vi "Page - Bank.vi"(8 "error in (no error)":errorcluster, 11 "Node Ptr":T1 format="%.0x") -> (0 "error out":errorcluster)   [LabVIEW 2015, in "SLSC-12201 DIO System Explorer.lvlib"]
uses:
  SLSC-12201 DIO System Explorer.lvlib
  <vilib>/NI Veristand/Custom Device API/Custom Device Item Ref.ctl
  Shared/Constants.vi
  <vilib>/NI Veristand/Custom Device API/Get Item Property (Boolean).vi
  <vilib>/NI Veristand/Custom Device API/Custom Device API.lvlib
  Shared/SLSC-12201 DIO Shared.lvlib
panel:
  in  "*Enable Pull-up Resistors":bool
  in  "*33V Input Threshold":dbl caption="Input Threshold"
  in  "*5V Input Threshold":dbl caption="Input Threshold"
  in  "*Enable 5V Range":bool
  in  "*Select Vsup":u16(ring) caption="Voltage Supply Selector" items=["Off", "Vsup_0", "Vsup_1"]
  in  "SHDocVw.IWebBrowser2":refnum<k7>(container)
  in  "Header":cluster{"Section Name":string}={"Section Name"="Custom Device Item Settings"}
  in  "Description":string
  out "Name":string
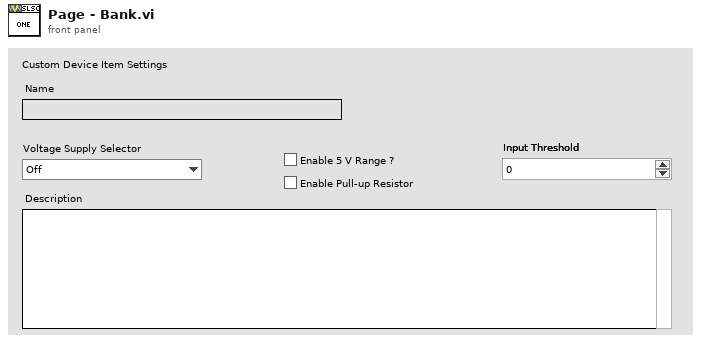
[diagram p1: front panel]
types:
  T1 = typedef "Custom Device API.lvlib/Custom Device Item Ref.ctl" = u64
  T2 = typedef "Custom Device API.lvlib/Custom Device Item Info.ctl" = cluster{"Name":string, "Is Channel":bool, "GUID":string, "Is Waveform":bool}
  T3 = typedef "Custom Device API.lvlib/Custom Device Channel.ctl" = cluster{"Type":T4, "Units":string, "Default Value":dbl, "Faultable":bool, "Scalable":bool}
  T4 = typedef "Custom Device API.lvlib/Custom Device Channel Type.ctl" = enum16{"Input", "Output"}
  T5 = cluster{"Channel Name":string, "SLSC Name":string, "Channel":T3}[]
  T6 = typedef "Custom Device API.lvlib/Custom Device Commands.ctl" = enum16{"Default", "Item renamed", "Shutdown", "Dynamic button pressed"}
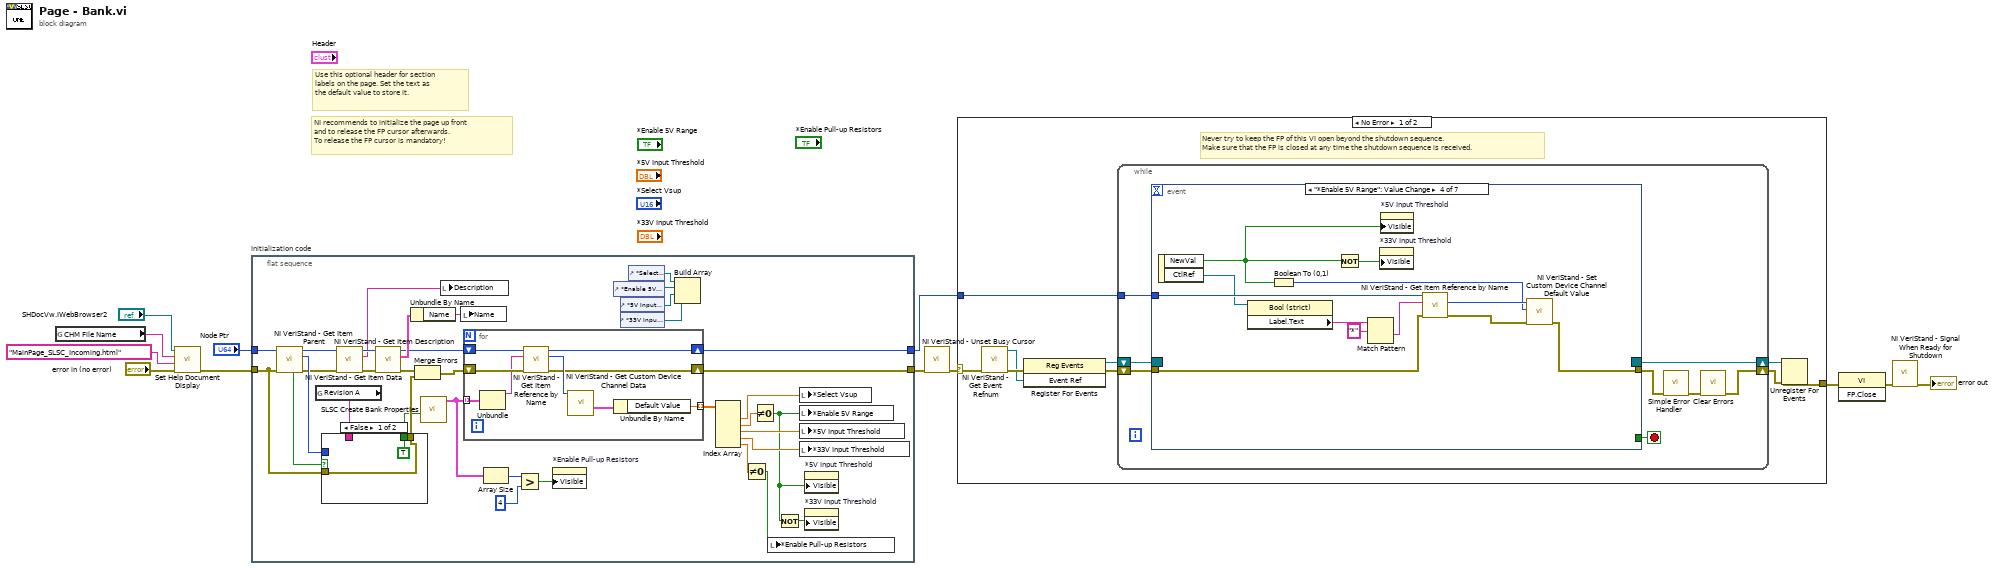
[diagram p0: block diagram]
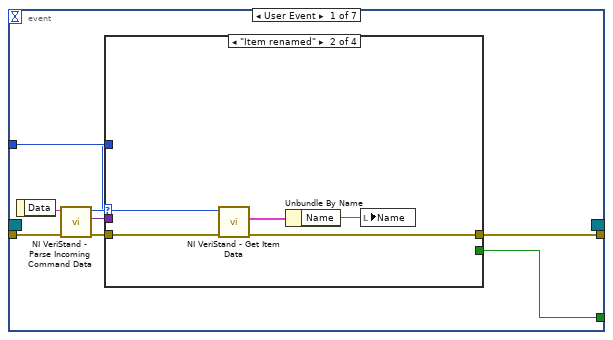
[diagram p2: hidden frame]
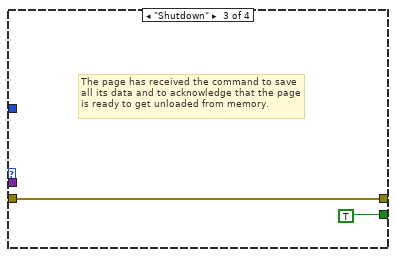
[diagram p4: hidden frame]
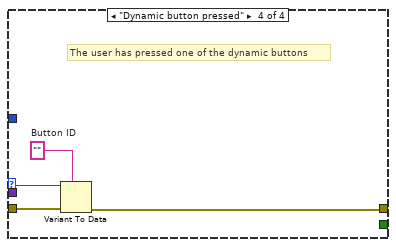
[diagram p5: hidden frame]
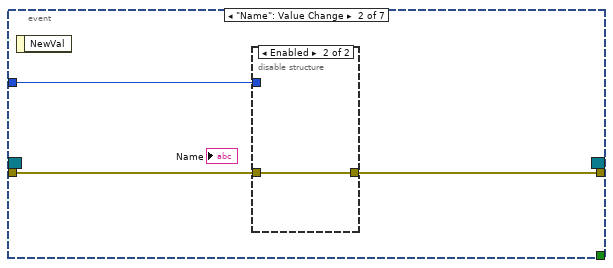
[diagram p6: hidden frame]
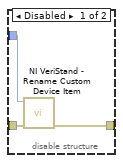
[diagram p7: hidden frame]
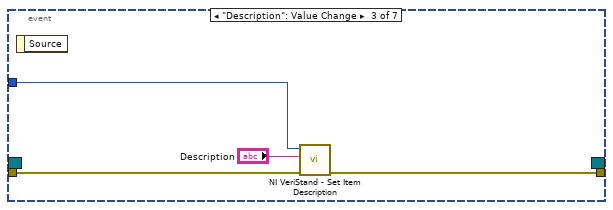
[diagram p8: hidden frame]
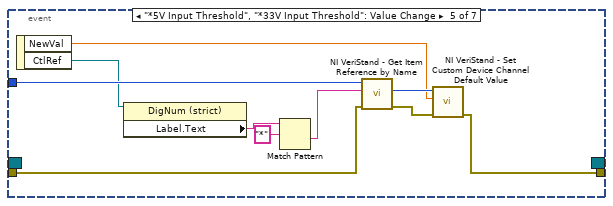
[diagram p9: hidden frame]
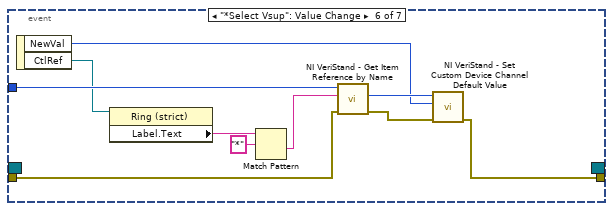
[diagram p10: hidden frame]
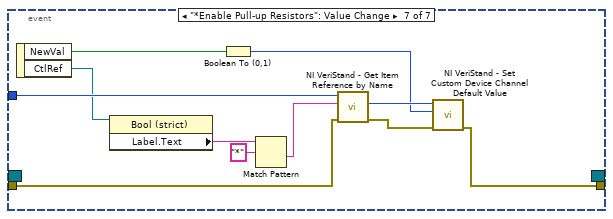
[diagram p11: hidden frame]
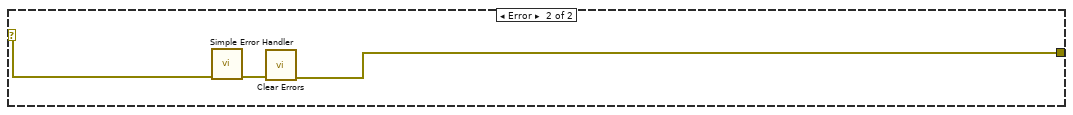
[diagram p12: hidden frame]
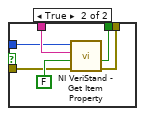
[diagram p13: hidden frame]
diagram:
  # "Use this optional header for section labels on the page. Set the text as the default value to store it."
  # "NI recommends to initialize the page up front\nand to release the FP cursor afterwards.\nTo release the FP cursor is mandatory!"
  n1 = global read "Constants.vi" "CHM File Name"() -> (w1:string)
  n2 = call "Set Help Document Display.vi"("error in (no error)"="error in (no error)", "HTML File"="MainPage_SLSC_Incoming.html", "Main CHM File"=w1, "SHDocVw.IWebBrowser2"="SHDocVw.IWebBrowser2") -> ("error out"=w2:errorcluster)  [unwired: 7 in]
  n3 = flat-sequence "Initialization code" {
    tunnel: w2 -> [w18]
    tunnel: "Node Ptr" -> [w21]
    tunnel: [w42] -> w8
    tunnel: [w40] -> w6
    frame #0 {
      n4 = call <vilib>:"NI VeriStand - Get Item Parent.vi"("error in (no error)"=w18, "Item Ref in"=w21) -> ("error out"=w17:errorcluster, "Parent Ref"=w19:T1, "Item Ref out"=w20:T1, "Found"=w13:bool)  [unwired: 6 in]
      n5 = global read "Constants.vi" "Revision A"() -> (w22:string)
      n6 = case shown="False" w13 {
        tunnel: w22 -> [_ w55]
        tunnel: w19 -> [_ w54]
        tunnel: w18 -> [w49 w53]
        tunnel: [w49 w52] -> w15
        tunnel: [TRUE ("Value") w51] -> w14
        frame False {
        }
        frame True {
          n7 = call-poly <vilib>:"NI VeriStand - Get Item Property.vi"("error in (no error)"=w53, "Default Value"=FALSE, "Property Name"=w55, "Item Ref in"=w54) -> ("error out"=w52:errorcluster, "Value"=w51:bool)  [unwired: 4 in, 2 out]
        }
      }
      n8 = call <vilib>:"NI VeriStand - Get Item Description.vi"("error in (no error)"=w17, "Item Ref in"=w20) -> ("error out"=w46:errorcluster, "Description"=w47:string, "Item Ref out"=w48:T1)  [unwired: 7 out]
      n9 = call <vilib>:"NI VeriStand - Get Item Data.vi"("error in (no error)"=w46, "Item Ref in"=w48) -> ("error out"=w43:errorcluster, "Item Info"=w45:T2, "Item Ref out"=w41:T1)  [unwired: 7 out]
      n10 = Unbundle By Name(w45) -> ("Name"=w44:string)
      n11 = Merge Errors(w43, w15) -> (w16:errorcluster)
      n12 = call "SLSC Create Bank Properties.vi"("RevA?"=w14) -> ("Outgoing configuration"=w28:T5)  [unwired: 10 in]
      n13 = local write "Description"(w47) -> ()
      n14 = local write "Name"(w44) -> ()
      n15 = for {
        shift-right: [w62] -> w42
        shift-left: w16 -> [w63]
        shift-right: [w60] -> w40
        shift-left: w41 -> [w61]
        tunnel: w28 -> [w59] mode=indexing
        tunnel: [w57] -> w35 mode=indexing
        n16 = Unbundle(w59) -> ("Channel Name"=w58:string)  [unwired: 2 out]
        n17 = call <vilib>:"NI VeriStand - Get Item Reference by Name.vi"("error in (no error)"=w63, "Item Name"=w58, "Parent Ref in"=w61) -> ("error out"=w62:errorcluster, "Item Ref"=w65:T1, "Parent Ref out"=w60:T1)  [unwired: 5 in, 1 out]
        n18 = call <vilib>:"NI VeriStand - Get Custom Device Channel Data.vi"("Channel Ref in"=w65) -> ("Channel"=w64:T3)  [unwired: 5 in, 5 out]
        n19 = Unbundle By Name(w64) -> ("Default Value"=w57:dbl)
      }
      n20 = Array Size(array=w28) -> (size(s)=w27:i32)
      n21 = Greater?(x=w27, y=4) -> (0:w25:bool)
      n22 = property on="*Enable Pull-up Resistors" class="Bool (strict)"("Visible"=w25) -> ()  [unwired: 2 in, 2 out]
      n23 = control-ref of="*Enable 5V Range"() -> (w38:refnum<vi>)
      n24 = control-ref of="*5V Input Threshold"() -> (w37:refnum<vi>)
      n25 = control-ref of="*33V Input Threshold"() -> (w36:refnum<vi>)
      n26 = control-ref of="*Select Vsup"() -> (w39:refnum<vi>)
      n27 = Build Array(w39, w38, w37, w36) -> ()  [unwired: 1 out]
      n28 = Index Array(array=w35) -> (element #1=w34:dbl, element #2=w33:dbl, element #3=w31:dbl, element #4=w32:dbl, element #5=w24:dbl)  [unwired: 5 in]
      n29 = Not Equal To 0?(x=w24) -> (x != 0?=w23:bool)
      n30 = Not Equal To 0?(x=w33) -> (x != 0?=w29:bool)
      n31 = local write "*Enable Pull-up Resistors"(w23) -> ()
      n32 = Not(x=w29) -> (.not. x?=w30:bool)
      n33 = local write "*Select Vsup"(w34) -> ()
      n34 = local write "*Enable 5V Range"(w29) -> ()
      n35 = local write "*5V Input Threshold"(w31) -> ()
      n36 = local write "*33V Input Threshold"(w32) -> ()
      n37 = property on="*5V Input Threshold" class="DigNum (strict)"("Visible"=w29) -> ()  [unwired: 2 in, 2 out]
      n38 = property on="*33V Input Threshold" class="DigNum (strict)"("Visible"=w30) -> ()  [unwired: 2 in, 2 out]
    }
  }
  n39 = call <vilib>:"NI VeriStand - Unset Busy Cursor.vi"("error in (no error)"=w8) -> ("error out"=w7:errorcluster)  [unwired: 10 out]
  n40 = case shown="No Error" w7 {
    selector: w7 -> [w66 w159]
    tunnel: [w71 w157] -> w12
    tunnel: w6 -> [w67 _]
    frame No Error {
      # "Never try to keep the FP of this VI open beyond the shutdown sequence.\nMake sure that the FP is closed at any time the shutdown sequence is received."
      n41 = call <vilib>:"NI VeriStand - Get Event Refnum.vi"("error in (no error)"=w66) -> ("error out"=w74:errorcluster, "Event Ref"=w70:refnum<user-event>)  [unwired: 9 out]
      n42 = register-events(error in=w74, w70) -> (reference out=w68:refnum<event-registration>, error out=w69:errorcluster)  [unwired: 1 in]
      n43 = while {
        tunnel: w67 -> [w78]
        shift-right: [w75] -> w72
        shift-left: w69 -> [w81]
        shift-right: [w82] -> w73
        shift-left: w68 -> [w80]
        stop <- w79 stop-if-true
        n44 = event shown="[3] \"*Enable 5V Range\": Value Change" {
          selector: w80 -> [_ _ _ _ _ _ _]
          dyn-events: [_ _ _ _ _ _ _] -> w82
          timeout: _ -> [_ _ _ _ _ _ _]
          tunnel: w81 -> [w90 w105 w112 w122 w133 w143 w154]
          tunnel: [w86 _ _ _ _ _ _] -> w79
          tunnel: [w85 w104 w111 w120 w131 w141 w152] -> w77
          tunnel: w78 -> [w84 w103 w113 w125 w135 w145 w156]
          event User Event {
            n45 = event-data() -> ("Data"=w89:string)  [unwired: 1 out]
            n46 = call <vilib>:"NI VeriStand - Parse Incoming Command Data.vi"("error in (no error)"=w90, "Incoming data"=w89) -> ("error out"=w88:errorcluster, "Outgoing data"=w83:variant, "Action"=w87:T6)  [unwired: 7 out]
            n47 = case shown="\"Item renamed\"" w87 {
              tunnel: w88 -> [w91 w96 w97 w102]
              tunnel: [_ _ TRUE _] -> w86
              tunnel: [w91 w93 w97 w99] -> w85
              tunnel: w84 -> [_ w95 _ _]
              tunnel: w83 -> [_ _ _ w101]
              frame "Default", Default {
              }
              frame "Item renamed" {
                n48 = call <vilib>:"NI VeriStand - Get Item Data.vi"("error in (no error)"=w96, "Item Ref in"=w95) -> ("error out"=w93:errorcluster, "Item Info"=w94:T2)  [unwired: 8 out]
                n49 = Unbundle By Name(w94) -> ("Name"=w92:string)
                n50 = local write "Name"(w92) -> ()
              }
              frame "Shutdown" {
                # "The page has received the command to save all its data and to acknowledge that the page is ready to get unloaded from memory."
              }
              frame "Dynamic button pressed" {
                w100 = ""  # Button ID
                # "The user has pressed one of the dynamic buttons"
                n51 = Variant To Data(error in=w102, type=w100, Variant=w101) -> (error out=w99:errorcluster)  [unwired: 1 out]
              }
            }
          }
          event "Name": Value Change {
            n52 = event-data() -> ()  [unwired: 2 out]
            n53 = disable-structure shown="Enabled" {
              disable-tunnel: w105 -> [w108 w109]
              disable-tunnel: [w107 w109] -> w104
              disable-tunnel: w103 -> [w106 _]
              frame Disabled {
                n54 = call <vilib>:"NI VeriStand - Rename Custom Device Item.vi"("error in (no error)"=w108, "Item Ref in"=w106) -> ("error out"=w107:errorcluster)  [unwired: 2 in, 7 out]
              }
              frame Enabled {
              }
            }
          }
          event "Description": Value Change {
            n55 = event-data() -> ()  [unwired: 2 out]
            n56 = call <vilib>:"NI VeriStand - Set Item Description.vi"("error in (no error)"=w112, "Description"="Description", "Item Ref in"=w113) -> ("error out"=w111:errorcluster)  [unwired: 8 out]
          }
          event "*Enable 5V Range": Value Change {
            n57 = event-data() -> ("NewVal"=w114:bool, "CtlRef"=w117:refnum<vi>)  [unwired: 1 out]
            n58 = property class="Bool (strict)"(reference=w117) -> ("Label.Text"=w119:string)  [unwired: 1 in, 2 out]
            n59 = Boolean To (0,1)(Boolean=w114) -> (0, 1=w123:i16)
            n60 = Not(x=w114) -> (.not. x?=w115:bool)
            n61 = Match Pattern(string=w119, regular expression="*") -> (after substring=w116:string)  [unwired: 1 in, 3 out]
            n62 = property on="*33V Input Threshold" class="DigNum (strict)"("Visible"=w115) -> ()  [unwired: 2 in, 2 out]
            n63 = property on="*5V Input Threshold" class="DigNum (strict)"("Visible"=w114) -> ()  [unwired: 2 in, 2 out]
            n64 = call <vilib>:"NI VeriStand - Get Item Reference by Name.vi"("error in (no error)"=w122, "Item Name"=w116, "Parent Ref in"=w125) -> ("error out"=w121:errorcluster, "Item Ref"=w124:T1)  [unwired: 5 in, 2 out]
            n65 = call <vilib>:"NI VeriStand - Set Custom Device Channel Default Value.vi"("error in (no error)"=w121, "Default Value"=w123, "Channel Ref in"=w124) -> ("error out"=w120:errorcluster)  [unwired: 7 in, 1 out]
          }
          event "*5V Input Threshold", "*33V Input Threshold": Value Change {
            n66 = event-data() -> ("NewVal"=w130:dbl, "CtlRef"=w126:refnum<vi>)  [unwired: 1 out]
            n67 = property class="DigNum (strict)"(reference=w126) -> ("Label.Text"=w129:string)  [unwired: 1 in, 2 out]
            n68 = Match Pattern(string=w129, regular expression="*") -> (after substring=w127:string)  [unwired: 1 in, 3 out]
            n69 = call <vilib>:"NI VeriStand - Get Item Reference by Name.vi"("error in (no error)"=w133, "Item Name"=w127, "Parent Ref in"=w135) -> ("error out"=w132:errorcluster, "Item Ref"=w134:T1)  [unwired: 5 in, 2 out]
            n70 = call <vilib>:"NI VeriStand - Set Custom Device Channel Default Value.vi"("error in (no error)"=w132, "Default Value"=w130, "Channel Ref in"=w134) -> ("error out"=w131:errorcluster)  [unwired: 7 in, 1 out]
          }
          event "*Select Vsup": Value Change {
            n71 = event-data() -> ("NewVal"=w136:u16, "CtlRef"=w140:refnum<vi>)  [unwired: 1 out]
            n72 = property class="Ring (strict)"(reference=w140) -> ("Label.Text"=w139:string)  [unwired: 1 in, 2 out]
            n73 = Match Pattern(string=w139, regular expression="*") -> (after substring=w137:string)  [unwired: 1 in, 3 out]
            n74 = call <vilib>:"NI VeriStand - Get Item Reference by Name.vi"("error in (no error)"=w143, "Item Name"=w137, "Parent Ref in"=w145) -> ("error out"=w142:errorcluster, "Item Ref"=w144:T1)  [unwired: 5 in, 2 out]
            n75 = call <vilib>:"NI VeriStand - Set Custom Device Channel Default Value.vi"("error in (no error)"=w142, "Default Value"=w136, "Channel Ref in"=w144) -> ("error out"=w141:errorcluster)  [unwired: 7 in, 1 out]
          }
          event "*Enable Pull-up Resistors": Value Change {
            n76 = event-data() -> ("NewVal"=w147:bool, "CtlRef"=w151:refnum<vi>)  [unwired: 1 out]
            n77 = property class="Bool (strict)"(reference=w151) -> ("Label.Text"=w150:string)  [unwired: 1 in, 2 out]
            n78 = Boolean To (0,1)(Boolean=w147) -> (0, 1=w146:i16)
            n79 = Match Pattern(string=w150, regular expression="*") -> (after substring=w148:string)  [unwired: 1 in, 3 out]
            n80 = call <vilib>:"NI VeriStand - Get Item Reference by Name.vi"("error in (no error)"=w154, "Item Name"=w148, "Parent Ref in"=w156) -> ("error out"=w153:errorcluster, "Item Ref"=w155:T1)  [unwired: 5 in, 2 out]
            n81 = call <vilib>:"NI VeriStand - Set Custom Device Channel Default Value.vi"("error in (no error)"=w153, "Default Value"=w146, "Channel Ref in"=w155) -> ("error out"=w152:errorcluster)  [unwired: 7 in, 1 out]
          }
        }
        n82 = call <vilib>:"Simple Error Handler.vi"("error in (no error)"=w77) -> ("error out"=w76:errorcluster)  [unwired: 1 in, 7 out]
        n83 = call <vilib>:"Clear Errors.vi"("error in (no error)"=w76) -> ("error out"=w75:errorcluster)  [unwired: 1 in, 5 out]
      }
      n84 = Unregister For Events(event registration refnum=w73, error in=w72) -> (error out=w71:errorcluster)
    }
    frame Error {
      n85 = call <vilib>:"Simple Error Handler.vi"("error in (no error)"=w159) -> ("error out"=w158:errorcluster)  [unwired: 1 in, 7 out]
      n86 = call <vilib>:"Clear Errors.vi"("error in (no error)"=w158) -> ("error out"=w157:errorcluster)  [unwired: 1 in, 5 out]
    }
  }
  n87 = invoke class="VI" method="FP.Close"(error in=w12) -> (error out=w11:errorcluster)  [unwired: 2 in, 2 out]
  n88 = call <vilib>:"NI VeriStand - Signal When Ready for Shutdown.vi"("error in (no error)"=w11) -> ("error out"=→"error out":errorcluster)  [unwired: 10 out]
